vi "RunningAverager.vi"(8 "Reset":bool, 9 "n":i32, 11 "Input":dbl) -> (3 "Output":dbl)   [LabVIEW 2014]
uses:
  <vilib>/Analysis/baseanly.llb/Mean (DBL).vi
  <vilib>/Analysis/NI_AALBase.lvlib
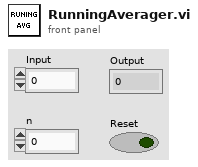
[diagram p1: front panel]
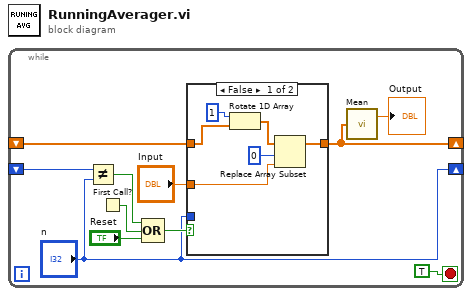
[diagram p0: block diagram]
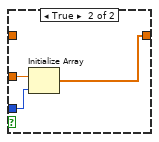
[diagram p2: hidden frame]
diagram:
  n1 = while {
    shift-right: [w9] -> _
    shift-left: _ -> [w10]
    shift-right: ["n"] -> _
    shift-left: _ -> [w4]
    stop <- TRUE stop-if-true
    n2 = Not Equal?(x=w4, y="n") -> (x != y?=w3:bool)
    n3 = First Call?() -> (First Call?: T/F=w2:bool)
    n4 = Compound Arithmetic op=OR(w3, w2, "Reset") -> (w6:bool)
    n5 = case shown="False" w6 {
      tunnel: "n" -> [_ w20]
      tunnel: "Input" -> [w12 w19]
      tunnel: [w17 w18] -> w9
      tunnel: w10 -> [w16 _]
      frame False {
        n6 = Rotate 1D Array(1:w16, 2:1 ("n")) -> (0:w15:dbl[])
        n7 = Replace Array Subset(array=w15, new element=w12, index=0) -> (w17:dbl[])
      }
      frame True {
        n8 = Initialize Array "Initialize Array"(w19, w20) -> (w18:dbl[])
      }
    }
    n9 = call-poly <vilib>:"Mean.vi"("X"=w9) -> ("mean"=→"Output":dbl)  [unwired: 1 out]
  }
